vi "login.vi"(0 "卡号":string, 1 "密码":string, 2 "文件":path=path "C:/Users/idea/Desktop/labview/名单.csv") -> (3 "匹配":bool, 5 "匹配信息":string[](array[string]), 6 "索引":i32)   [LabVIEW 2018]
uses:
  <vilib>/Utility/file.llb/Read Delimited Spreadsheet (string).vi
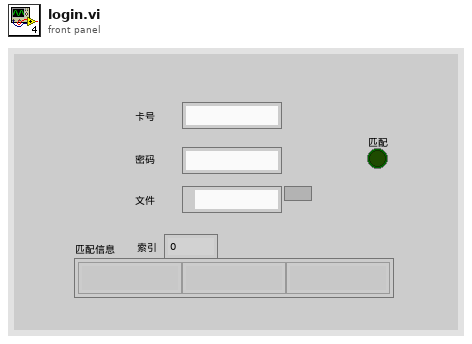
[diagram p1: front panel]
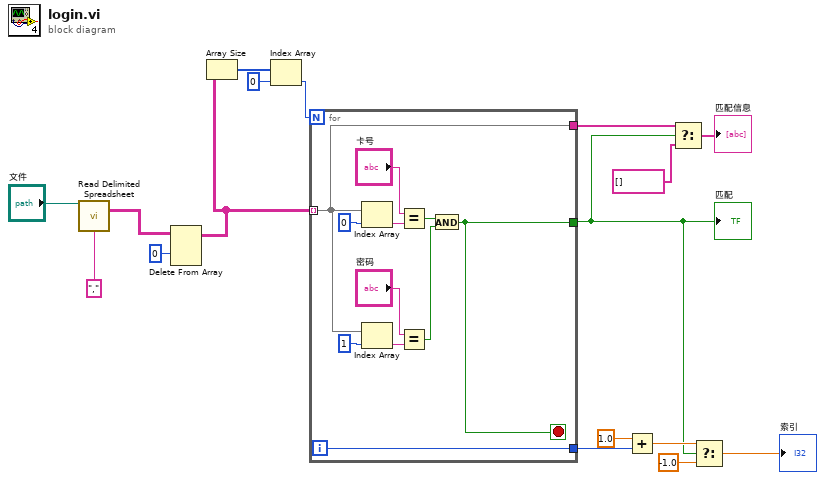
[diagram p0: block diagram]
diagram:
  n1 = call-poly <vilib>:"Read Delimited Spreadsheet.vi"("file path (dialog if empty)"="文件", "delimiter (\\t)"="," ("delimiter (\\t)")) -> ("all rows"=w15:string[][])  [unwired: 8 in, 5 out]
  n2 = Delete From Array(array=w15, index (row)=0 ("索引 (行)")) -> (array with subset deleted=w13:string[][])  [unwired: 2 in, 1 out]
  n3 = Array Size(array=w13) -> (size(s)=w11:i32[])
  n4 = Index Array(array=w11, index=0 ("索引")) -> (element=w12:i32)
  n5 = for {
    N: w12 -> [_]
    tunnel: w13 -> [w19] mode=indexing
    tunnel: [w20] -> w3
    tunnel: [w19] -> w9
    tunnel: [w18] -> w5
    i -> [w18]
    stop <- w20 stop-if-true
    n6 = Index Array(array=w19, index=0 ("索引")) -> (element=w26:string)
    n7 = Index Array(array=w19, index=1 ("索引")) -> (element=w23:string)
    n8 = Equal?(x="卡号", y=w26) -> (x = y?=w22:bool)
    n9 = Equal?(x="密码", y=w23) -> (x = y?=w21:bool)
    n10 = And(x=w22, y=w21) -> (x .and. y?=w20:bool)
  }
  "匹配" <- w3
  n11 = Add(x=1.0, y=w5) -> (x+y=w4:dbl)
  n12 = Select(t=w9, s=w3, f=string[] []) -> (s? t:f=→"匹配信息":string[])
  n13 = Select(t=w4, s=w3, f=-1.0) -> (s? t:f=→"索引":dbl)
